vi "auto_standup.vi"(1 "Angle":dbl, 2 "Encoder":dbl) -> (0 "PWM":dbl)   [LabVIEW 2018]
uses:
  Global_variables.vi
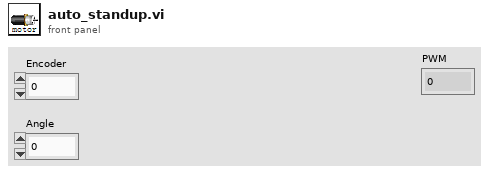
[diagram p1: front panel]
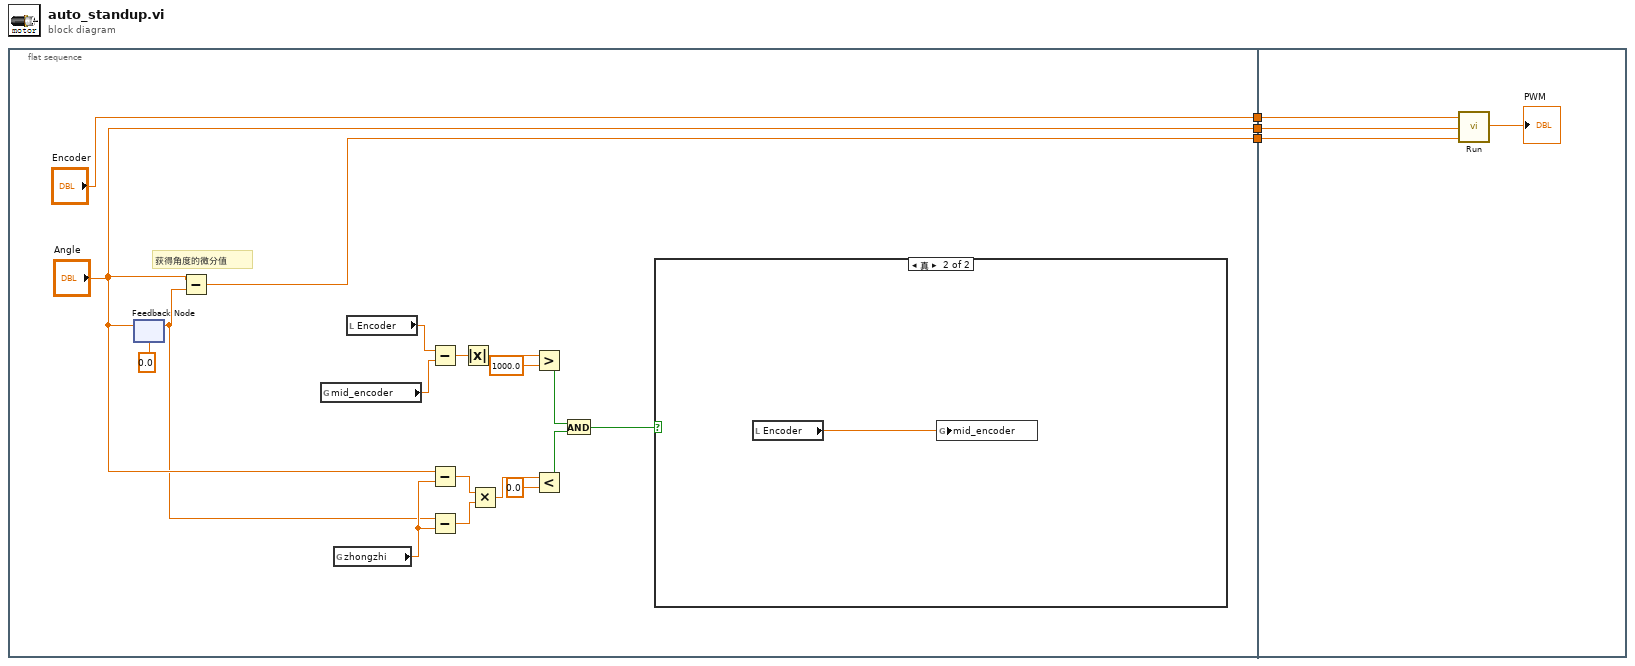
[diagram p0: block diagram]
diagram:
  n1 = flat-sequence {
    tunnel: ["Encoder"] -> w3
    tunnel: [w19] -> w2
    tunnel: ["Angle"] -> w1
    tunnel: w3 -> [w23]
    tunnel: w2 -> [w25]
    tunnel: w1 -> [w24]
    frame #0 {
      # "获得角度的微分值"
      n2 = feedback #1(0.0 ("Angle")) -> (w11:dbl)
      n3 = feedback-in #1("Angle") -> ()
      n4 = Subtract(x="Angle", y=w11) -> (x-y=w19:dbl)
      n5 = global read "Global_variables.vi" "mid_encoder"() -> (w18:dbl)
      n6 = global read "Global_variables.vi" "zhongzhi"() -> (w13:dbl)
      n7 = local read "Encoder"() -> (w17:dbl)
      n8 = Subtract(x=w17, y=w18) -> (x-y=w16:dbl)
      n9 = Subtract(x="Angle", y=w13) -> (x-y=w10:dbl)
      n10 = Subtract(x=w11, y=w13) -> (x-y=w9:dbl)
      n11 = Absolute Value(x=w16) -> (abs(x)=w15:dbl)
      n12 = Multiply(x=w10, y=w9) -> (x*y=w8:dbl)
      n13 = Greater?(x=w15, y=1000.0) -> (0:w6:bool)
      n14 = Less?(x=w8, y=0.0) -> (x < y?=w5:bool)
      n15 = And(x=w6, y=w5) -> (x .and. y?=w4:bool)
      n16 = case shown="真" w4 {
        frame False {
        }
        frame True {
          n17 = local read "Encoder"() -> (w22:dbl)
          n18 = global write "Global_variables.vi" "mid_encoder"(w22) -> ()
        }
      }
    }
    frame #1 {
      n19 = call "Run.vi"("D_Angle"=w25, "Angle"=w24, "Encoder"=w23) -> ("PWM"=→"PWM":dbl)  [unwired: 1 in]
    }
  }
